vi "Merge Directories__ogtk.vi"(6 "Ignore Read-Only? (FALSE)":bool, 7 "Delete Source? (FALSE)":bool, 8 "error in (no error)":errorcluster, 9 "Overwrite Existing Files? (FALSE)":bool, 10 "target directory path":path, 11 "source directory path":path) -> (0 "error out":errorcluster, 3 "dup target directory path":path)   [LabVIEW 2012]
doc: "Copies the contents of source directory into the destination directory. If source directory has subdirectories they will be copied into the destination directory recursively. Optionally, existing files may be overwritten, by setting the \"Overwrite Existing Files?\" input to TRUE. If you attempt to overwrite an existing file without setting to TRUE ans error will be returned. If FALSE, existing files will not be overwritten and no error wil be returned, Optionally, read-only files may be overwritten, by setting the \"Ignore Read-Only?\" input to TRUE. If you attempt to overwrite a read-only files without setting to TRUE an error will be returned. Optionally, by setting the \"Delete Source?\" input to TRUE the source directory will be deleted upon merge completion if no errors occured."
uses:
  <userlib>/_OpenG.lib/file/file.llb/Build Path - File Names Array__ogtk.vi
  <userlib>/_OpenG.lib/file/file.llb/Compare Two Paths - Scalar__ogtk.vi
  <userlib>/_OpenG.lib/file/file.llb/Build Path - Traditional - path__ogtk.vi
  <userlib>/_OpenG.lib/file/file.llb/Strip Path - Traditional__ogtk.vi
panel:
  # "OpenG Library.vi\n\nMerge Directories.vi\n\nCopies the contents of source directory into the destination directory.\n\nPlease visit http://www.OpenG.org to learn about the\nOpen Source LabVIEW software movement.\n\nNOTICE -- YOU MUST LEAVE THIS NOTICE IN PLACE.  PER THE TERMS OF THE LICENSE BELOW, YOU MAY SUBLICENSE THIS SOFTWARE \nIN ANY WAY THAT DOES NOT CONFLICT WITH THIS LICENSE.\n\n### BSD License (http://www.opensource.org/licenses/bsd-license.php) Begin ###\n \nCopyright (c) 2002-2004, Jim Kring <jim@jimkring.com>\nCopyright (c) 2002, Cal-Bay Systems, Inc. <info@calbay.com>\n\nAll rights reserved.\n\nRedistribution and use in source and binary forms, with or without modification, are permitted provided that the following conditions are met:\n\n    * Redistributions of source code must retain the above copyright notice, this list of conditions and the following disclaimer.\n    * Redistributions in binary form must reproduce the above copyright notice, this list of conditions and the following disclaimer in the \n       documentation and/or other materials provided with the distribution.\n    * Neither the name of SciWare, James Kring, Inc., nor the names of its contributors may be used to endorse or promote products derived \n       from this software without specific prior written permission.\n\nTHIS SOFTWARE IS PROVIDED BY THE COPYRIGHT HOLDERS AND CONTRIBUTORS \"AS IS\" AND ANY EXPRESS OR IMPLIED WARRANTIES, \nINCLUDING, BUT NOT LIMITED TO, THE IMPLIED WARRANTIES OF MERCHANTABILITY AND FITNESS FOR A PARTICULAR PURPOSE ARE \nDISCLAIMED. IN NO EVENT SHALL THE COPYRIGHT OWNER OR CONTRIBUTORS BE LIABLE FOR ANY DIRECT, INDIRECT, INCIDENTAL,\n SPECIAL, EXEMPLARY, OR CONSEQUENTIAL DAMAGES (INCLUDING, BUT NOT LIMITED TO, PROCUREMENT OF SUBSTITUTE GOODS OR \nSERVICES; LOSS OF USE, DATA, OR PROFITS; OR BUSINESS INTERRUPTION) HOWEVER CAUSED AND ON ANY THEORY OF LIABILITY, \nWHETHER IN CONTRACT, STRICT LIABILITY, OR TORT (INCLUDING NEGLIGENCE OR OTHERWISE) ARISING IN ANY WAY OUT OF THE USE \nOF THIS SOFTWARE, EVEN IF ADVISED OF THE POSSIBILITY OF SUCH DAMAGE.\n\n### BSD License End ###"
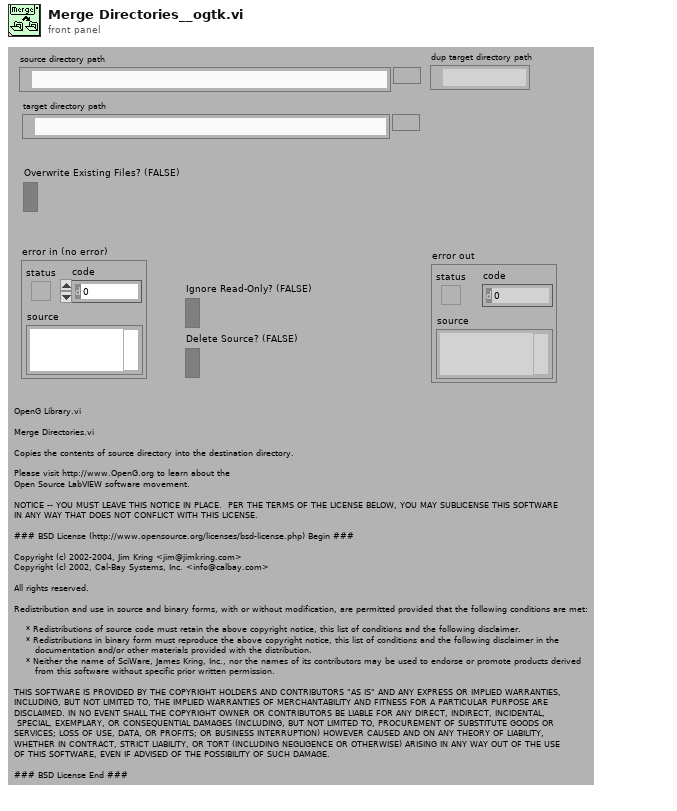
[diagram p1: front panel]
types:
  T1 = cluster{"Archive":bool, "Normal":bool, "Temporary":bool, "Compressed":bool, "Offline":bool, "Content Indexed":bool, "Encrypted (cannot set)":bool}
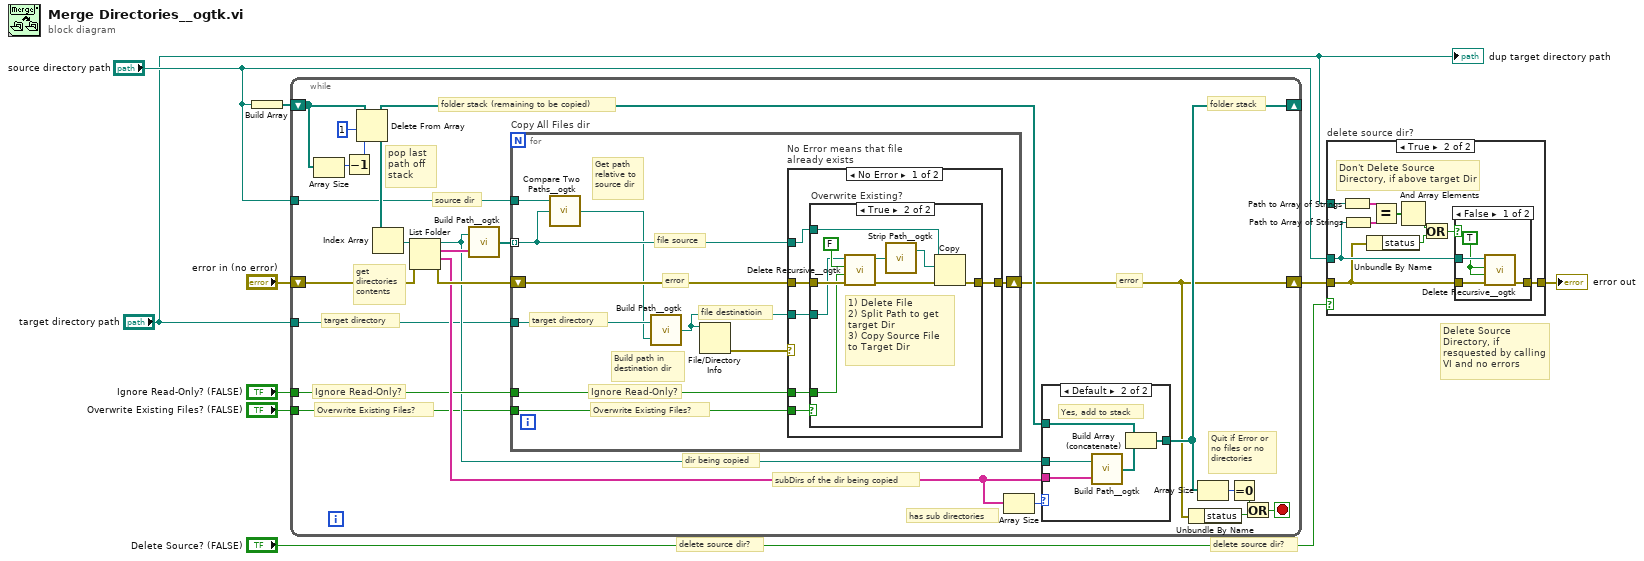
[diagram p0: block diagram]
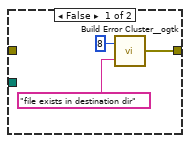
[diagram p3: hidden frame]
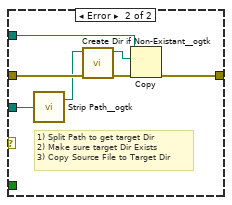
[diagram p4: hidden frame]
diagram:
  # "Delete Source Directory, if resquested by calling VI and no errors"
  # "delete source dir?"
  # "delete source dir?"
  n1 = Build Array("source directory path") -> (w8:path[])
  n2 = while {
    shift-right: [w18] -> _
    shift-left: w8 -> [w21]
    shift-right: [w10] -> w5
    shift-left: "error in (no error)" -> [w22]
    tunnel: "Ignore Read-Only? (FALSE)" -> [w17]
    tunnel: "source directory path" -> [w13]
    tunnel: "target directory path" -> [w12]
    tunnel: "Overwrite Existing Files? (FALSE)" -> [w11]
    stop <- w23 stop-if-true
    (unwired) T1 {"Archive"=FALSE, "Normal"=FALSE, "Temporary"=FALSE, "Compressed"=FALSE, "Offline"=FALSE, "Content Indexed"=FALSE, "Encrypted (cannot set)"=FALSE} ("FileAttribute")
    # "folder stack"
    # "error"
    # "Overwrite Existing Files?"
    # "Ignore Read-Only?"
    # "target directory"
    # "subDirs of the dir being copied"
    # "dir being copied"
    # "folder stack (remaining to be copied)"
    # "source dir"
    # "get directories contents"
    # "pop last path off stack"
    # "Quit if Error or no files or no directories"
    # "has sub directories"
    n3 = Array Size(array=w21) -> (size(s)=w19:i32)
    n4 = Decrement(x=w19) -> (x-1=w20:i32)
    n5 = Delete From Array(array=w21, length=1 ("Length"), index=w20) -> (deleted portion=w32:path[], array with subset deleted=w27:path[])
    n6 = Index Array(array=w32) -> (element=w31:path)  [unwired: 1 in]
    n7 = List Folder(path=w31, error in=w22) -> (path out=w15:path, filenames=w16:string[], folder names=w28:string[], error out=w30:errorcluster)  [unwired: 2 in]
    n8 = call-poly <userlib>:"Build Path__ogtk.vi"("name or relative path"=w16, "base path"=w15) -> ("appended path"=w14:path[])
    n9 = for "Copy All Files dir" {
      shift-right: [w45] -> w10
      shift-left: w30 -> [w46]
      tunnel: w17 -> [w43]
      tunnel: w14 -> [w41] mode=indexing
      tunnel: w13 -> [w42]
      tunnel: w12 -> [w49]
      tunnel: w11 -> [w44]
      # "Ignore Read-Only?"
      # "Overwrite Existing Files?"
      # "file destinatioin"
      # "file source"
      # "target directory"
      # "error"
      # "Build path in destination dir"
      # "Get path relative to source dir"
      n10 = call-poly <userlib>:"Compare Two Paths__ogtk.vi"("path2"=w41, "path1"=w42) -> ("relative path from 1 to 2"=w40:path)  [unwired: 1 in, 2 out]
      n11 = call-poly <userlib>:"Build Path__ogtk.vi"("name or relative path"=w40, "base path"=w49) -> ("appended path"=w47:path)
      n12 = File/Directory Info(path=w47) -> (error out=w48:errorcluster)  [unwired: 1 in, 6 out]
      n13 = case "No Error means that file\nalready exists" shown="No Error" w48 {
        tunnel: w47 -> [w52 w72]
        tunnel: w41 -> [w51 w74]
        tunnel: w46 -> [w54 w71]
        tunnel: [w53 w73] -> w45
        tunnel: w44 -> [w55 _]
        tunnel: w43 -> [w50 _]
        frame No Error {
          n14 = case "Overwrite Existing?" shown="True" w55 {
            tunnel: w54 -> [_ w67]
            tunnel: [w56 w65] -> w53
            tunnel: w52 -> [_ w61]
            tunnel: w51 -> [_ w64]
            tunnel: w50 -> [_ w63]
            frame False {
              n15 = call <userlib>:"Build Error Cluster__ogtk.vi"("String to Prepend to source (\"\")"="file exists in destination dir" ("String to Prepend to source (\"\")"), "code"=8) -> ("error out"=w56:errorcluster)
            }
            frame True {
              # "1) Delete File\n2) Split Path to get target Dir\n3) Copy Source File to Target Dir"
              n16 = call <userlib>:"Delete Recursive__ogtk.vi"("error in (no error)"=w67, "Ignore Read-Only? (FALSE)"=w63, "Recursive? (FALSE)"=FALSE, "Path"=w61) -> ("error out"=w66:errorcluster, "dup Path"=w60:path)  [unwired: 6 in]
              n17 = call-poly <userlib>:"Strip Path__ogtk.vi"("path"=w60) -> ("stripped path"=w59:path)  [unwired: 1 out]
              n18 = Copy(8:w66, 10:w59, 11:w64) -> (0:w65:errorcluster)  [unwired: 2 in, 2 out]
            }
          }
        }
        frame Error {
          # "1) Split Path to get target Dir\n2) Make sure target Dir Exists\n3) Copy Source File to Target Dir"
          n19 = call-poly <userlib>:"Strip Path__ogtk.vi"("path"=w72) -> ("stripped path"=w68:path)  [unwired: 1 out]
          n20 = call <userlib>:"Create Dir if Non-Existant__ogtk.vi"("error in (no error)"=w71, "Directory Path"=w68) -> ("error out"=w70:errorcluster, "dup Directory Path"=w69:path)  [unwired: 7 in, 1 out]
          n21 = Copy(8:w70, 10:w69, 11:w74) -> (0:w73:errorcluster)  [unwired: 2 in, 2 out]
        }
      }
    }
    n22 = Array Size(array=w28) -> (size(s)=w29:i32)
    n23 = case shown="Default" w29 {
      tunnel: w15 -> [_ w35]
      tunnel: w28 -> [_ w39]
      tunnel: w27 -> [w34 w37]
      tunnel: [w34 w36] -> w18
      frame 0 {
      }
      frame Default {
        # "Yes, add to stack"
        n24 = call-poly <userlib>:"Build Path__ogtk.vi"("name or relative path"=w39, "base path"=w35) -> ("appended path"=w38:path[])
        n25 = Build Array (concatenate)(w37, w38) -> (w36:path[])
      }
    }
    n26 = Unbundle By Name(w10) -> ("status"=w25:bool)
    n27 = Array Size(array=w18) -> (size(s)=w26:i32)
    n28 = Equal To 0?(x=w26) -> (x = 0?=w24:bool)
    n29 = Or(x=w24, y=w25) -> (x .or. y?=w23:bool)
  }
  n30 = case "delete source dir?" shown="True" "Delete Source? (FALSE)" {
    tunnel: w5 -> [w75 w79]
    tunnel: [w75 w85] -> w4
    tunnel: "source directory path" -> [_ w83]
    tunnel: "target directory path" -> [_ w84]
    frame False {
    }
    frame True {
      # "Don't Delete Source Directory, if above target Dir"
      n31 = Path to Array of Strings(0:w84) -> (2:w82:string[])  [unwired: 1 out]
      n32 = Path to Array of Strings(0:w83) -> (2:w81:string[])  [unwired: 1 out]
      n33 = Unbundle By Name(w79) -> ("status"=w76:bool)
      n34 = Equal?(x=w82, y=w81) -> (x = y?=w80:bool[])
      n35 = And Array Elements(Boolean array=w80) -> (logical AND=w78:bool)
      n36 = Or(x=w78, y=w76) -> (x .or. y?=w77:bool)
      n37 = case shown="False" w77 {
        tunnel: w83 -> [w89 _]
        tunnel: [w88 w90] -> w85
        tunnel: w79 -> [w86 w90]
        frame False {
          w87 = TRUE
          n38 = call <userlib>:"Delete Recursive__ogtk.vi"("error in (no error)"=w86, "Ignore Read-Only? (FALSE)"=w87, "Recursive? (FALSE)"=w87, "Path"=w89) -> ("error out"=w88:errorcluster)  [unwired: 6 in, 1 out]
        }
        frame True {
        }
      }
    }
  }
  "error out" <- w4
  "dup target directory path" <- "target directory path"
